vi "Configure Serial Bus (Flexray - Autosetup).vi"(0 "VISA resource name":refnum<visa-resource-name>, 5 "Serial Bus Name (1: Serial Bus 1)":i32(ring)=1 items=["Serial Bus 1"=1, "Serial Bus 2"=2], 11 "error in (no error)":errorcluster) -> (4 "VISA resource name out":refnum<visa-resource-name>, 15 "error out":errorcluster)   [LabVIEW 2017, in "Agilent 2000 3000 X-Series.lvlib"]
doc: "Configures oscilloscope settings to facilitate FlexRay triggering and serial decode automatically.\n\nSets the selected source channel's impedance to 50 Ohms.\nSets the selected source channel' s probe attenuation to 10:1.\nSets the trigger level (on the selected source channel) to - 300 mV.\nTurns on trigger Noise Reject.\nTurns on Serial Decode.\nSets the trigger to the specified serial bus.\n\nNote:\nThis VI is not supported by EDUX1052A/G, DSOX1202A/G, DSOX1204A/G models"
uses:
  Agilent 2000 3000 X-Series.lvlib
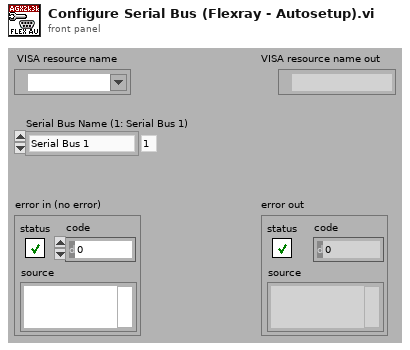
[diagram p1: front panel]
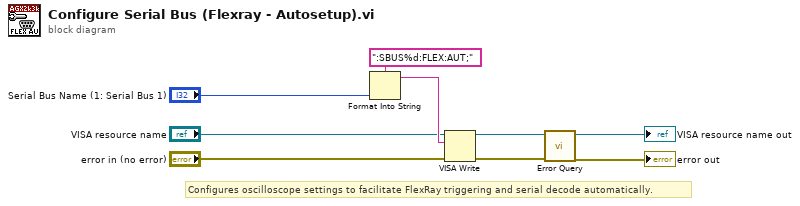
[diagram p0: block diagram]
diagram:
  # "Configures oscilloscope settings to facilitate FlexRay triggering and serial decode automatically."
  n1 = Format Into String(format string=":SBUS%d:FLEX:AUT;", "Serial Bus Name (1: Serial Bus 1)") -> (resulting string=w7:string)  [unwired: 2 in, 1 out]
  n2 = VISA Write(VISA resource name="VISA resource name", write buffer=w7, error in (no error)="error in (no error)") -> (VISA resource name out=w4:refnum<visa-resource-name>, error out=w3:errorcluster)  [unwired: 1 out]
  n3 = call "Error Query.vi"("error in (no error)"=w3, "VISA resource name"=w4) -> ("error out"=→"error out":errorcluster, "VISA resource name out"=→"VISA resource name out":refnum<visa-resource-name>)  [unwired: 8 out]
